vi "test_BuildAdvancedAssets_TargetsDifferentCompilers.vi"() -> (3 "Pass?":bool)   [LabVIEW 2019, in "Tests.SolutionBuilder.lvlib"]
uses:
  Tests.SolutionBuilder.lvlib
  SolutionBuilder/SolutionBuilder.lvclass
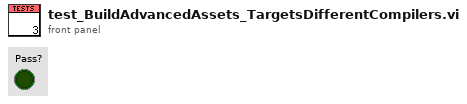
[diagram p1: front panel]
types:
  T1 = typedef "SolutionBuilder.lvlib/BuildManager.lvclass/GeneratedFile.ctl" = map{cluster{"Project path":string, "Build spec name":string}, set{string}}
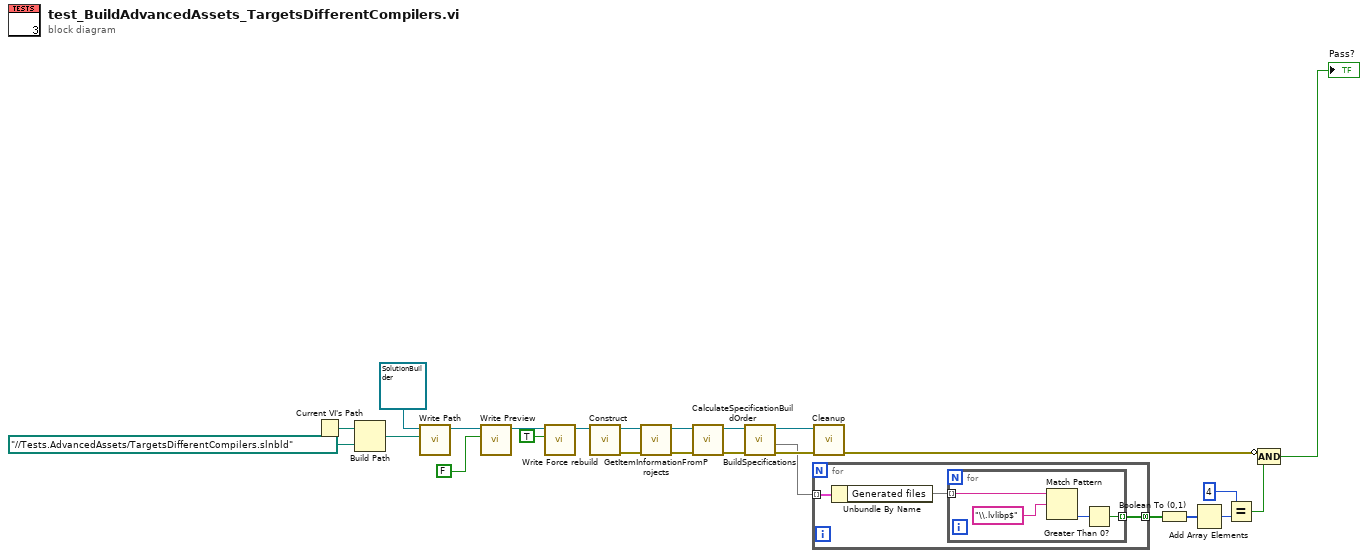
[diagram p0: block diagram]
diagram:
  n1 = Current VI's Path() -> (path=w24:path)
  n2 = Build Path(base path=w24, name or relative path=path "../../Tests.AdvancedAssets/TargetsDifferentCompilers.slnbld" ("Path")) -> (appended path=w22:path)
  n3 = call "Write Path.vi"("Path"=w22, "SolutionBuilder in"=refnum<class "SolutionBuilder.lvclass"> refnum) -> ("SolutionBuilder out"=w13:refnum<class "SolutionBuilder.lvclass">)  [unwired: 9 in]
  n4 = call "Write Preview.vi"("Preview?"=FALSE, "SolutionBuilder in"=w13) -> ("SolutionBuilder out"=w3:refnum<class "SolutionBuilder.lvclass">)  [unwired: 9 in]
  n5 = call "Write Force rebuild.vi"("Force rebuild"=TRUE, "SolutionBuilder in"=w3) -> ("SolutionBuilder out"=w2:refnum<class "SolutionBuilder.lvclass">)  [unwired: 9 in]
  n6 = call "Construct.vi"("SolutionBuilder in"=w2) -> ("error out"=w18:errorcluster, "SolutionBuilder out"=w21:refnum<class "SolutionBuilder.lvclass">)  [unwired: 9 in]
  n7 = call "GetItemInformationFromProjects.vi"("error in (no error)"=w18, "SolutionBuilder in"=w21) -> ("error out"=w17:errorcluster, "SolutionBuilder out"=w20:refnum<class "SolutionBuilder.lvclass">)  [unwired: 8 in]
  n8 = call "CalculateSpecificationBuildOrder.vi"("error in (no error)"=w17, "SolutionBuilder in"=w20) -> ("error out"=w16:errorcluster, "SolutionBuilder out"=w19:refnum<class "SolutionBuilder.lvclass">)  [unwired: 8 in]
  n9 = call "BuildSpecifications.vi"("error in (no error)"=w16, "SolutionBuilder in"=w19) -> ("error out"=w15:errorcluster, "Generated file"=w5:T1, "SolutionBuilder out"=w14:refnum<class "SolutionBuilder.lvclass">)  [unwired: 7 in]
  n10 = for {
    tunnel: w5 -> [w28] mode=indexing
    tunnel: [w26] -> w10 mode=concatenating
    n11 = Unbundle By Name(w28) -> ("Generated files"=w27:set{string})
    n12 = for {
      tunnel: w27 -> [w29] mode=indexing
      tunnel: [w30] -> w26 mode=indexing
      n13 = Match Pattern(string=w29, regular expression="\\.lvlibp$") -> (offset past match=w31:i32)  [unwired: 1 in, 3 out]
      n14 = Greater Than 0?(x=w31) -> (x > 0?=w30:bool)
    }
  }
  n15 = call "Cleanup.vi"("error in (no error)"=w15, "SolutionBuilder in"=w14) -> ("error out"=w11:errorcluster)  [unwired: 8 in, 1 out]
  n16 = Boolean To (0,1)(Boolean=w10) -> (0, 1=w7:i16[])
  n17 = Add Array Elements(numeric array=w7) -> (sum=w6:i16)
  n18 = Equal?(x=i16 4, y=w6) -> (x = y?=w8:bool)
  n19 = Compound Arithmetic op=AND(invert w11, w8) -> (→"Pass?":bool)
